vi "Get HP Data.vi"(8 "Clust Refnum":refnum<vi>, 11 "HP Chosen Data Type":string) -> (0 "error out":errorcluster, 3 "ControlRefNums":refnum<vi>[](array[refnum]))   [LabVIEW 2016, in "M1M3SupportEUI_Views.lvlib"]
uses:
  M1M3SupportEUI_Views.lvlib
  Typedefs/HP Events.ctl
  SALLV_m1m3/DataTypes/logevent_HardpointActuatorInfo.ctl
  SALLV_m1m3/DataTypes/logevent_HardpointActuatorState.ctl
  SALLV_m1m3/DataTypes/logevent_HardpointActuatorWarning.ctl
  SALLV_m1m3/DataTypes/logevent_HardpointMonitorInfo.ctl
  SALLV_m1m3/DataTypes/logevent_HardpointMonitorState.ctl
  SALLV_m1m3/DataTypes/logevent_HardpointMonitorWarning.ctl
  SALLV_m1m3/SALLV_m1m3.lvlib
  Typedefs/M1M3SupportEUI_TypeDefs.lvlib
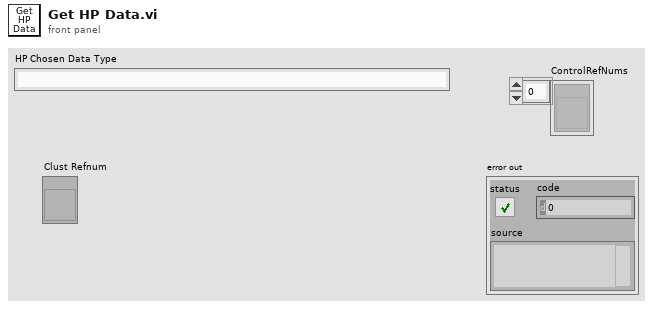
[diagram p1: front panel]
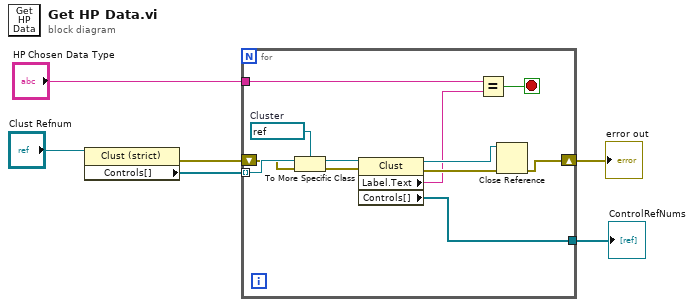
[diagram p0: block diagram]
diagram:
  n1 = property class="Clust (strict)"(reference="Clust Refnum") -> (error out=w4:errorcluster, "Controls[]"=w5:refnum<vi>[])  [unwired: 1 in, 1 out]
  n2 = for {
    tunnel: w5 -> [w18] mode=indexing
    shift-right: [w12] -> w2
    shift-left: w4 -> [w17]
    tunnel: "HP Chosen Data Type" -> [w8]
    tunnel: [w7] -> w1
    stop <- w10 stop-if-true
    w16 = refnum<vi> refnum  # Cluster
    n3 = To More Specific Class(target class=w16, reference=w18, error in=w17) -> (specific class reference=w15:refnum<vi>, error out=w14:errorcluster)
    n4 = property class="Clust"(reference=w15, error in=w14) -> (reference out=w11:refnum<vi>, error out=w13:errorcluster, "Label.Text"=w9:string, "Controls[]"=w7:refnum<vi>[])
    n5 = Equal?(x=w8, y=w9) -> (x = y?=w10:bool)
    n6 = Close Reference(reference=w11, error in (no error)=w13) -> (error out=w12:errorcluster)
  }
  "ControlRefNums" <- w1
  "error out" <- w2
